vi "Do.vi"(8 "error in (no error)":errorcluster, 10 "Actor in":refnum<class "Actor.lvclass">, 11 "WebSocket Server Enqueuer Msg":refnum<class "WebSocket Server Enqueuer Msg.lvclass">) -> (0 "error out":errorcluster, 2 "Actor out":refnum<class "Actor.lvclass">)   [LabVIEW 2016, in "Test Server Manager.lvlib" / "WebSocket Server Enqueuer Msg.lvclass"]
doc: "(<B>Filename</B>: Actor Framework.lvlib:Message.lvclass:Do.vi)\n\nDefines what a message does when it is received by an actor. Generally, a message instructs an actor to invoke one of its methods. By default, this method does nothing. A child class must override it to define behavior. Create a child class by using the Actor Framework Message Maker dialog box."
uses:
  WebSocket Server Enqueuer Msg.lvclass
  C:/Projects/Shared Libraries/WebSocket Actor/WebSocket Actor/Abstract Messages/WebSocket Server-Service Enqueuer Msg/WebSocket Server-Service Enqueuer Msg.lvclass
  <vilib>/ActorFramework/Actor/Actor.lvclass
  WS Test Server/WS Test Server.lvclass
  C:/Program Files (x86)/National Instruments/LabVIEW 2016/vi.lib/ActorFramework/Actor/Actor.lvclass
  WebSocket Actor/Abstract Messages/WebSocket Server-Service Enqueuer Msg/WebSocket Server-Service Enqueuer Msg.lvclass/WebSocket Server-Service Enqueuer Msg.ctl
  WS Test Server/WS Test Server.lvclass/WS Test Server.ctl
  WS Test Server/properties/Write WebSocket Server Enqueuer.vi
  WebSocket Actor/Abstract Messages/WebSocket Server-Service Enqueuer Msg/properties/Read WebSocket Service Enqueuer.vi
  WebSocket Actor/Abstract Messages/WebSocket Server-Service Enqueuer Msg/properties/Read Error .vi
  <vilib>/ActorFramework/Message Enqueuer/Message Enqueuer.lvclass
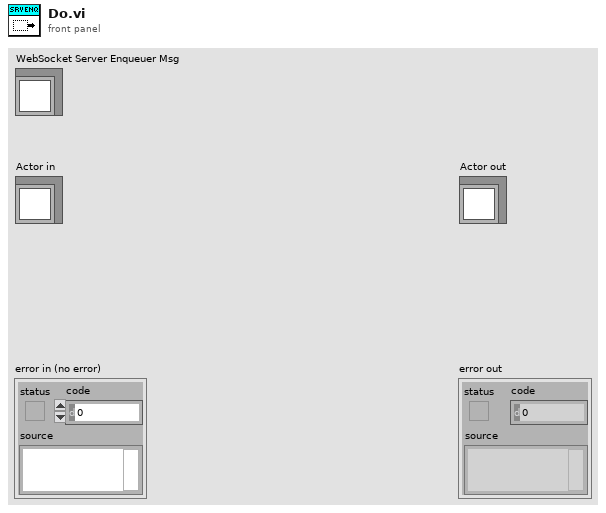
[diagram p1: front panel]
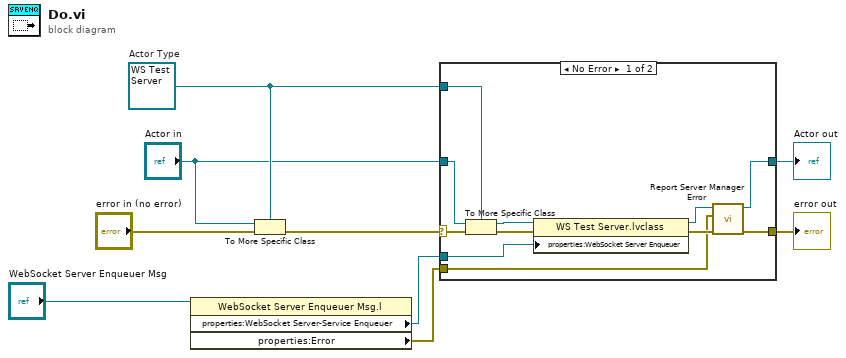
[diagram p0: block diagram]
diagram:
  w8 = refnum<class "WS Test Server.lvclass"> refnum  # Actor Type
  n1 = property class="WebSocket Server Enqueuer Msg.l"(reference="WebSocket Server Enqueuer Msg") -> ("properties:WebSocket Server-Service Enqueuer"=w2:refnum<class "Message Enqueuer.lvclass">, "properties:Error "=w1:errorcluster)  [unwired: 1 in, 2 out]
  n2 = To More Specific Class(target class=w8, reference="Actor in", error in="error in (no error)") -> (error out=w9:errorcluster)  [unwired: 1 out]
  n3 = case shown="No Error" w9 {
    selector: w9 -> [w20 w22]
    tunnel: [w12 w22] -> w4
    tunnel: [w10 w21] -> w5
    tunnel: "Actor in" -> [w19 w21]
    tunnel: w8 -> [w18 _]
    tunnel: w2 -> [w15 _]
    tunnel: w1 -> [w13 _]
    frame No Error {
      n4 = To More Specific Class ("Actor Cast")(target class=w18, reference=w19, error in=w20) -> (specific class reference=w17:refnum<class "WS Test Server.lvclass">, error out=w16:errorcluster)
      n5 = property class="WS Test Server.lvclass"(reference=w17, error in=w16, "properties:WebSocket Server Enqueuer"=w15) -> (reference out=w11:refnum<class "WS Test Server.lvclass">, error out=w14:errorcluster)
      n6 = call "Report Server Manager Error.vi"("error in (no error)"=w14, "Server Manager Error"=w13, "WS Test Server in"=w11) -> ("error out"=w12:errorcluster, "WS Test Server out"=w10:refnum<class "WS Test Server.lvclass">)  [unwired: 7 in]
    }
    frame Error {
    }
  }
  "error out" <- w4
  "Actor out" <- w5
